vi "loadTuner.vi"(0 "configuration file path":path=path "C:/users/develoer/desktop/foo.ini", 11 "error in (no error)":errorcluster) -> (4 "file path":path, 6 "hue":cluster{dbl, dbl}(slide)={0.0, 4.747474747474747} scale=0.0..10.0, 8 "sat":cluster{dbl, dbl}(slide)={0.0, 4.747474747474747} scale=0.0..10.0, 10 "val":cluster{dbl, dbl}(slide)={0.0, 4.747474747474747} scale=0.0..10.0, 15 "error out":errorcluster)   [LabVIEW 2016]
uses:
  <vilib>/Utility/config.llb/Read Key (Double).vi
  <vilib>/Utility/config.llb/NI_LVConfig.lvlib
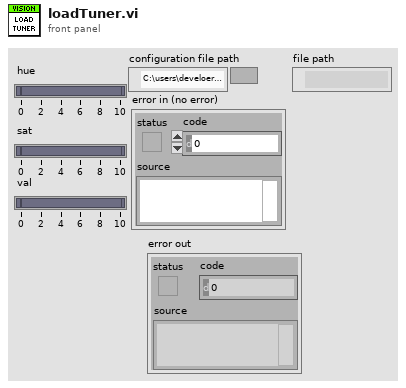
[diagram p1: front panel]
types:
  T1 = typedef "NI_LVConfig.lvlib/Config Data RefNum.ctl" = refnum<k1>
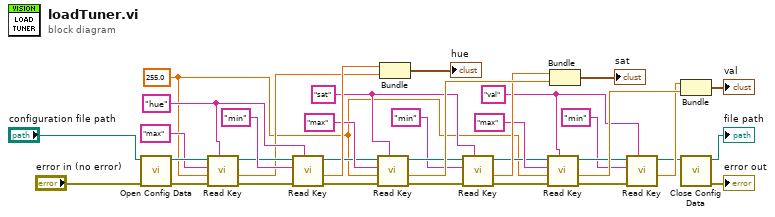
[diagram p0: block diagram]
diagram:
  w1 = 255.0 ("default value")
  w9 = "val" ("section")
  w19 = "sat" ("section")
  w32 = "hue" ("section")
  n1 = call <vilib>:"Open Config Data.vi"("error in (no error)"="error in (no error)", "configuration file path"="configuration file path") -> ("error out"=w30:errorcluster, "refnum"=w36:T1)  [unwired: 7 in, 1 out]
  n2 = call-poly <vilib>:"Read Key.vi"("section"=w32, "error in (no error)"=w30, "default value"=w1, "key"="max", "refnum"=w36) -> ("error out"=w29:errorcluster, "value"=w24:dbl, "refnum out"=w33:T1)  [unwired: 3 in, 1 out]
  n3 = call-poly <vilib>:"Read Key.vi"("section"=w32, "error in (no error)"=w29, "key"="min", "refnum"=w33) -> ("error out"=w14:errorcluster, "value"=w25:dbl, "refnum out"=w15:T1)  [unwired: 4 in, 1 out]
  n4 = call-poly <vilib>:"Read Key.vi"("section"=w19, "error in (no error)"=w14, "default value"=w1, "key"="max", "refnum"=w15) -> ("error out"=w20:errorcluster, "value"=w22:dbl, "refnum out"=w18:T1)  [unwired: 3 in, 1 out]
  n5 = Bundle("value"=w25, "value"=w24) -> (→"hue":cluster{"value":dbl, "value":dbl})  [unwired: 1 in]
  n6 = call-poly <vilib>:"Read Key.vi"("section"=w19, "error in (no error)"=w20, "key"="min", "refnum"=w18) -> ("error out"=w4:errorcluster, "value"=w21:dbl, "refnum out"=w5:T1)  [unwired: 4 in, 1 out]
  n7 = call-poly <vilib>:"Read Key.vi"("section"=w9, "error in (no error)"=w4, "default value"=w1, "key"="max", "refnum"=w5) -> ("error out"=w10:errorcluster, "value"=w12:dbl, "refnum out"=w8:T1)  [unwired: 3 in, 1 out]
  n8 = Bundle("value"=w21, "value"=w22) -> (→"sat":cluster{"value":dbl, "value":dbl})  [unwired: 1 in]
  n9 = call-poly <vilib>:"Read Key.vi"("section"=w9, "error in (no error)"=w10, "key"="min", "refnum"=w8) -> ("value"=w11:dbl, "refnum out"=w2:T1)  [unwired: 4 in, 2 out]
  n10 = Bundle("value"=w11, "value"=w12) -> (→"val":cluster{"value":dbl, "value":dbl})  [unwired: 1 in]
  n11 = call <vilib>:"Close Config Data.vi"("refnum"=w2) -> ("error out"=→"error out":errorcluster, "file path"=→"file path":path)  [unwired: 9 in]
